vi "combinational-logic-7-segment.vi"(8 "4-bit-reg-input":T1) -> (0 "4-bit-reg-output":T1, 3 "7-segment CTRL out":T2)   [LabVIEW 2021]
uses:
  controls/4-bit-disp.ctl
  controls/7-segment-display.ctl
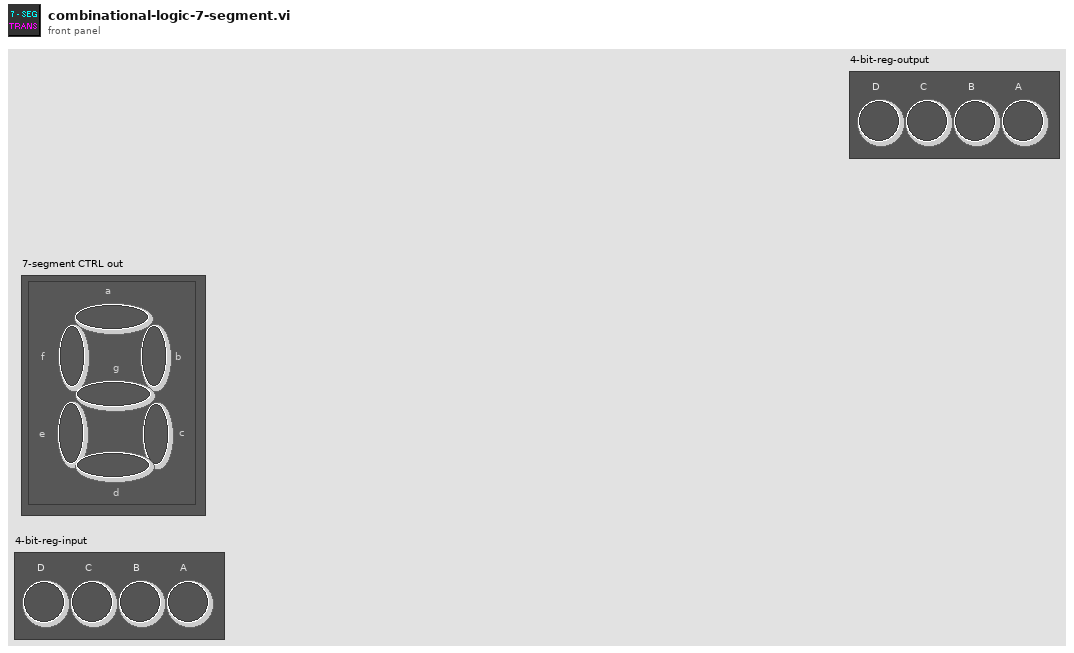
[diagram p1: front panel]
types:
  T1 = typedef "4-bit-disp.ctl" = cluster{"D":bool, "C":bool, "B":bool, "A":bool}
  T2 = typedef "7-segment-display.ctl" = cluster{"a":bool, "b":bool, "c":bool, "d":bool, "e":bool, "f":bool, "g":bool}
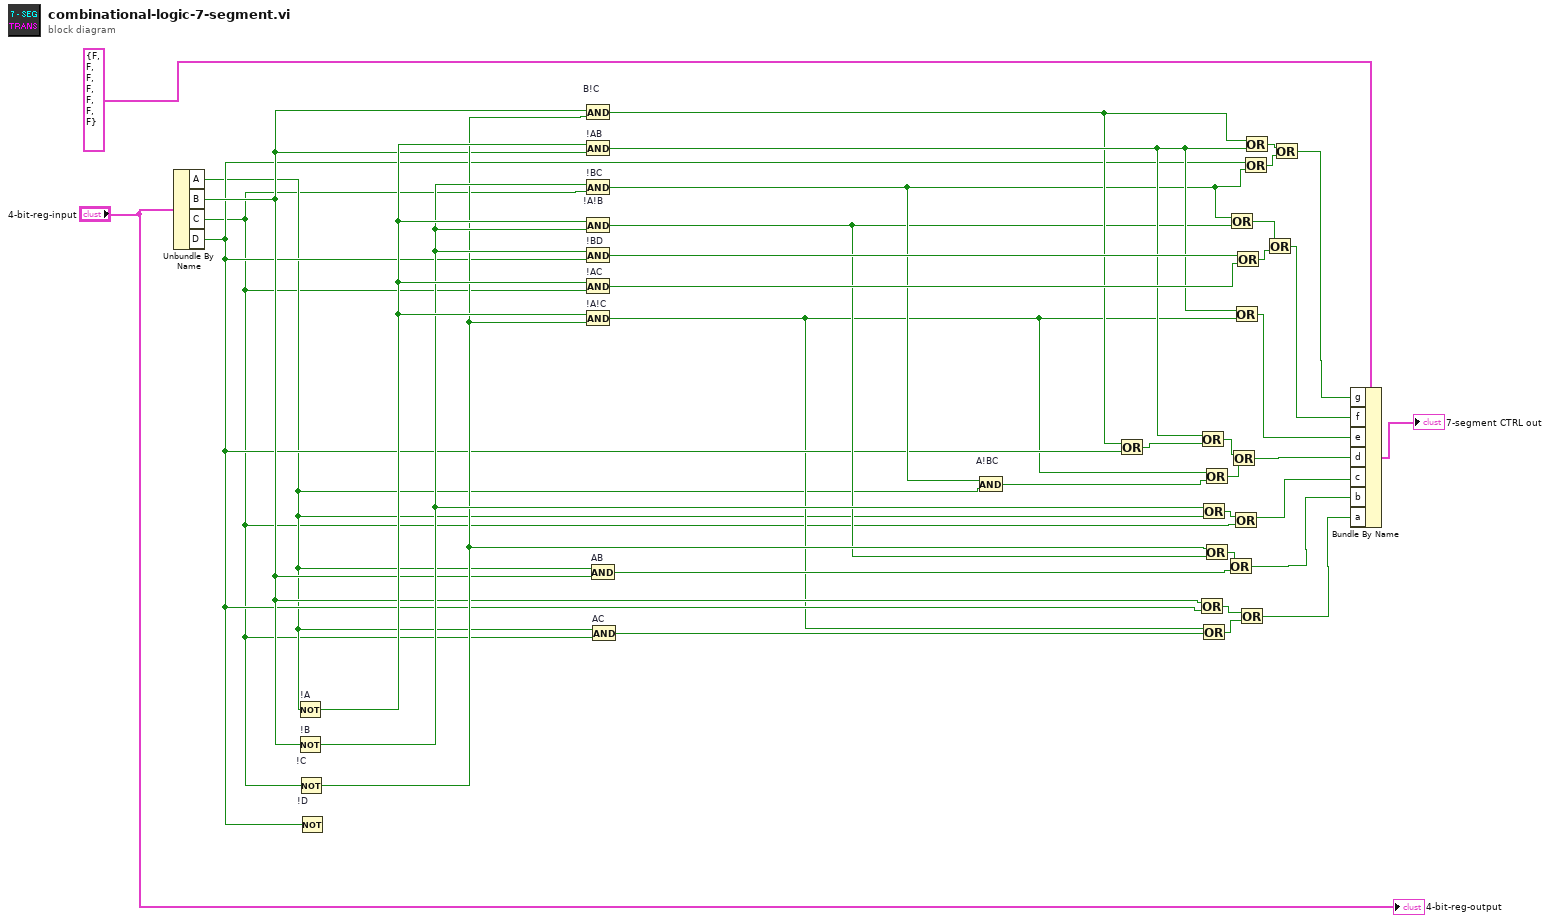
[diagram p0: block diagram]
diagram:
  n1 = Unbundle By Name("4-bit-reg-input") -> ("A"=w2:bool, "B"=w6:bool, "C"=w1:bool, "D"=w5:bool)
  n2 = Not "!A"(x=w2) -> (.not. x?=w16:bool)
  n3 = Not "!B"(x=w6) -> (.not. x?=w10:bool)
  n4 = Not "!C"(x=w1) -> (.not. x?=w9:bool)
  n5 = Not "!D"(x=w5) -> ()  [unwired: 1 out]
  n6 = And "B!C"(x=w6, y=w9) -> (x .and. y?=w13:bool)
  n7 = And "!AB"(x=w16, y=w6) -> (x .and. y?=w15:bool)
  n8 = And "!BC"(x=w10, y=w1) -> (x .and. y?=w11:bool)
  n9 = And "!A!B"(x=w16, y=w10) -> (x .and. y?=w8:bool)
  n10 = And "!BD"(x=w10, y=w5) -> (x .and. y?=w18:bool)
  n11 = And "!AC"(x=w16, y=w1) -> (x .and. y?=w17:bool)
  n12 = And "!A!C"(x=w16, y=w9) -> (x .and. y?=w4:bool)
  n13 = And "AB"(x=w2, y=w6) -> (x .and. y?=w7:bool)
  n14 = And "AC"(x=w2, y=w1) -> (x .and. y?=w3:bool)
  n15 = And "A!BC"(x=w11, y=w2) -> (x .and. y?=w12:bool)
  n16 = Or(x=w13, y=w5) -> (x .or. y?=w14:bool)
  n17 = Or(x=w6, y=w5) -> (x .or. y?=w27:bool)
  n18 = Or(x=w15, y=w14) -> (x .or. y?=w31:bool)
  n19 = Or(x=w10, y=w2) -> (x .or. y?=w23:bool)
  n20 = Or(x=w4, y=w3) -> (x .or. y?=w26:bool)
  n21 = Or(x=w4, y=w12) -> (x .or. y?=w24:bool)
  n22 = Or(x=w9, y=w8) -> (x .or. y?=w29:bool)
  n23 = Or(x=w29, y=w7) -> (x .or. y?=w22:bool)
  n24 = Or(x=w11, y=w8) -> (x .or. y?=w21:bool)
  n25 = Or(x=w31, y=w24) -> (x .or. y?=w32:bool)
  n26 = Or(x=w23, y=w1) -> (x .or. y?=w30:bool)
  n27 = Or(x=w15, y=w4) -> (x .or. y?=w33:bool)
  n28 = Or(x=w18, y=w17) -> (x .or. y?=w34:bool)
  n29 = Or(x=w27, y=w26) -> (x .or. y?=w28:bool)
  n30 = Or(x=w5, y=w11) -> (x .or. y?=w19:bool)
  n31 = Or(x=w13, y=w15) -> (x .or. y?=w20:bool)
  n32 = Or(x=w21, y=w34) -> (x .or. y?=w35:bool)
  n33 = Or(x=w20, y=w19) -> (x .or. y?=w36:bool)
  n34 = Bundle By Name(cluster=T2 {"a"=FALSE, "b"=FALSE, "c"=FALSE, "d"=FALSE, "e"=FALSE, "f"=FALSE, "g"=FALSE} ("7-seg-typedef"), "g"=w36, "f"=w35, "e"=w33, "d"=w32, "c"=w30, "b"=w22, "a"=w28) -> (→"7-segment CTRL out":T2)
  "4-bit-reg-output" <- "4-bit-reg-input"
